vi "WPI_Camera CGI Parse for Exposure.vi"(11 "String":string="fixed_indoor") -> (1 "Numeric":i32, 2 "enum":T1)   [LabVIEW 2017]
uses:
  <vilib>/Rock Robotics/WPI/Camera/WPI_CameraExposure Values.ctl
  <vilib>/Rock Robotics/WPI/Camera/WPI_CameraWhite Balance Values.ctl
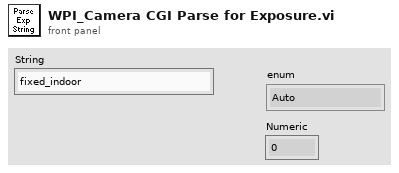
[diagram p1: front panel]
types:
  T1 = typedef "WPI_CameraExposure Values.ctl" = enum16{"Auto", "Flicker-free 50 Hz", "Flicker-free 60 Hz", "Hold current", "Custom"}
  T2 = typedef "WPI_CameraWhite Balance Values.ctl" = enum16{"Auto", "Fixed indoor", "Fixed outdoor 1", "Fixed outdoor 2", "Fixed fluorescent 1", "Fixed fluorescent 2", "Hold current", "Custom"}
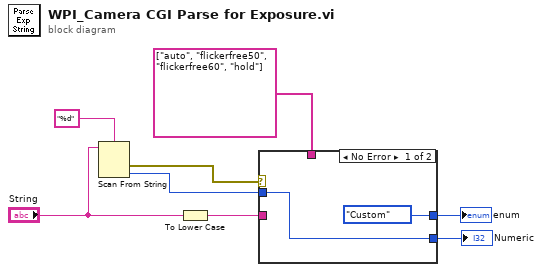
[diagram p0: block diagram]
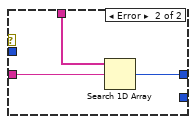
[diagram p2: hidden frame]
diagram:
  n1 = Scan From String(format string="%d", input string="String") -> (error out=w5:errorcluster, output 1=w3:i32)  [unwired: 3 in, 2 out]
  n2 = To Lower Case(string="String") -> (all lower case string=w8:string)
  n3 = case shown="No Error" w5 {
    tunnel: string[] ["auto", "flickerfree50", "flickerfree60", "hold"] -> [_ w13]
    tunnel: w8 -> [_ w12]
    tunnel: [WPI_CameraWhite_Balance_Values."Custom" ("enum") w11] -> w4
    tunnel: w3 -> [w10 _]
    tunnel: [w10 _] -> w2
    frame No Error {
    }
    frame Error {
      n4 = Search 1D Array(1D array=w13, element=w12) -> (index of element=w11:i32)  [unwired: 1 in]
    }
  }
  "enum" <- w4
  "Numeric" <- w2
